vi "Write.vi"(6 "high priority? (F)":bool, 7 "subchannel (0)":i32, 8 "abort (F)":bool, 9 "last element? (F)":bool, 10 "element":cluster{"cmd":string, "data":variant}, 11 "element valid? (T)":bool=TRUE) -> (0 "done?":bool, 2 "channel":T1)   [LabVIEW 2019, in "Event MessengerM.lvlib"]
uses:
  Event MessengerM.lvlib
  <vilib>/event_ctls.llb/usereventprio.ctl
  ChannelOp.ctl
  ))Channel.ctl
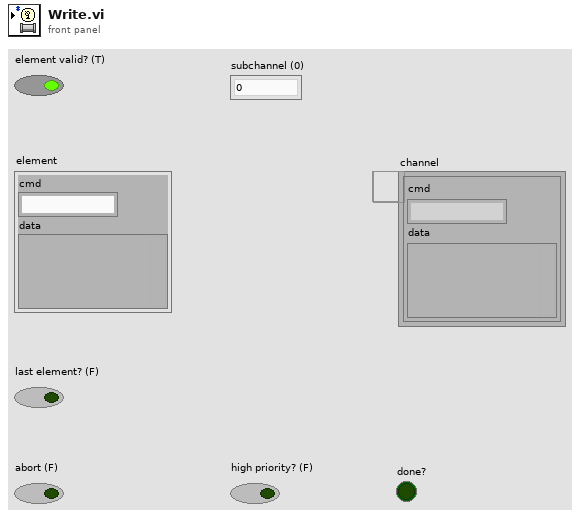
[diagram p1: front panel]
types:
  T1 = typedef "Event MessengerM.lvlib/))Channel.ctl" = refnum<queue>
  T2 = typedef "usereventprio.ctl" = enum32{"high priority", "normal priority"}
  T3 = typedef "Event MessengerM.lvlib/ChannelOp.ctl" = enum16{"init", "write", "register", "replicate", "probe"}
  T4 = cluster{"last element in":bool, "valid":bool, "abort in":bool, "event priority (norm)":T2}
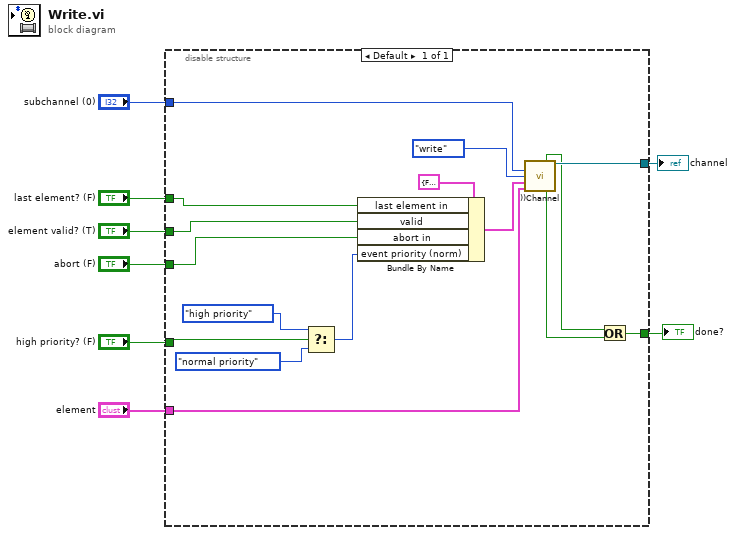
[diagram p0: block diagram]
diagram:
  n1 = disable-structure shown="Default" {
    disable-tunnel: "last element? (F)" -> [w15]
    disable-tunnel: "subchannel (0)" -> [w21]
    disable-tunnel: [w24] -> w1
    disable-tunnel: [w18] -> w2
    disable-tunnel: "element valid? (T)" -> [w16]
    disable-tunnel: "abort (F)" -> [w14]
    disable-tunnel: "high priority? (F)" -> [w13]
    disable-tunnel: "element" -> [w9]
    frame Enabled {
      n2 = Select(t=usereventprio."high priority" ("event priority (norm)"), s=w13, f=usereventprio."normal priority" ("event priority (normal)")) -> (s? t:f=w10:T2)
      n3 = Bundle By Name(cluster=T4 {"last element in"=FALSE, "valid"=FALSE, "abort in"=FALSE, "event priority (norm)"=enum."normal priority"} ("params"), "last element in"=w15, "valid"=w16, "abort in"=w14, "event priority (norm)"=w10) -> (w22:T4)
      n4 = call "))Channel.vi"("subchannel"=w21, "channelOp"=ChannelOp."write", "params"=w22, "element in"=w9) -> ("last element out"=w20:bool, "channel out"=w24:T1, "aborted?"=w19:bool)  [unwired: 7 in, 2 out]
      n5 = Or(x=w20, y=w19) -> (x .or. y?=w18:bool)
    }
  }
  "done?" <- w2
  "channel" <- w1
